vi "Messenger Initialize.vi"(7 "Elements Of Container":i32=-1, 8 "error in (no error)":errorcluster, 9 "Paras In 2":variant, 10 "Paras In":variant, 11 "Messenger Composite in":refnum<class "Simple Tree Queue Messenger.lvclass">) -> (0 "error out":errorcluster, 3 "Messenger Composite out":refnum<class "Simple Tree Queue Messenger.lvclass">)   [LabVIEW 2024, in "Simple Tree Queue Messenger.lvclass"]
uses:
  Simple Tree Queue Messenger.lvclass
  Ancestor Class/Message/Message.lvclass
  Simple Tree Queue Messenger.lvclass/Simple Tree Queue Messenger.ctl
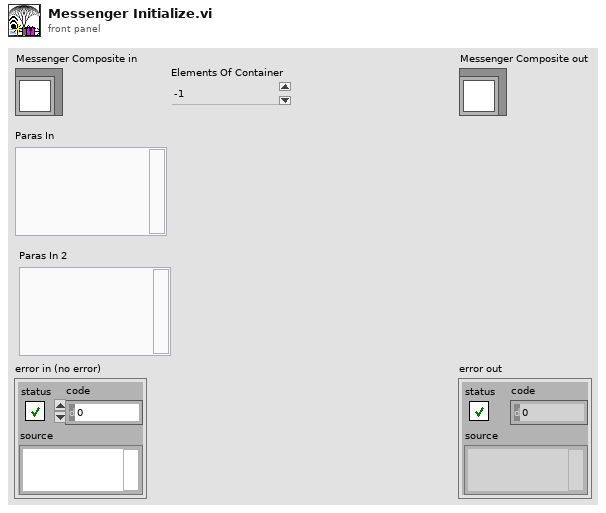
[diagram p1: front panel]
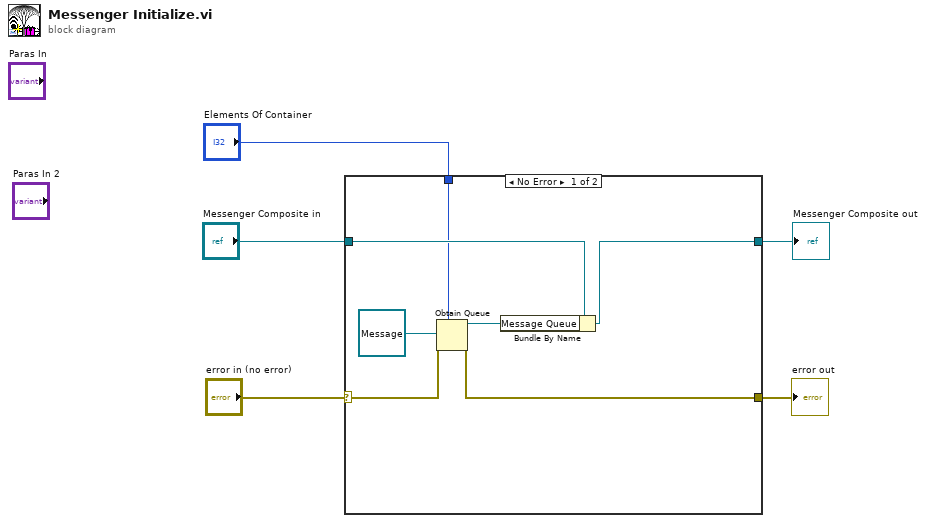
[diagram p0: block diagram]
diagram:
  n1 = case shown="No Error" "error in (no error)" {
    selector: "error in (no error)" -> [w9 w14]
    tunnel: [w8 w14] -> w4
    tunnel: [w10 w13] -> w3
    tunnel: "Messenger Composite in" -> [w11 w13]
    tunnel: "Elements Of Container" -> [w7 _]
    frame No Error {
      n2 = Obtain Queue(max queue size (-1, unlimited)=w7, element data type=refnum<class "Message.lvclass"> refnum ("Message.lvclass"), error in (no error)=w9) -> (queue out=w6:refnum<queue>, error out=w8:errorcluster)  [unwired: 2 in, 1 out]
      n3 = Bundle By Name(cluster=w11, "Message Queue"=w6) -> (w10:refnum<class "Simple Tree Queue Messenger.lvclass">)
    }
    frame Error {
    }
  }
  "error out" <- w4
  "Messenger Composite out" <- w3
